vi "Local Error Handler.vi"(6 "Clear? (T)":bool=TRUE, 7 "error in (no error)":errorcluster) -> (9 "error out":errorcluster)   [LabVIEW 2012, in "Win8uiFramework.lvlib"]
uses:
  <vilib>/Utility/error.llb/DialogType.ctl
  Win8uiFramework.lvlib
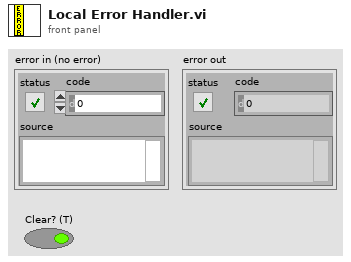
[diagram p1: front panel]
types:
  T1 = typedef "DialogType.ctl" = u16
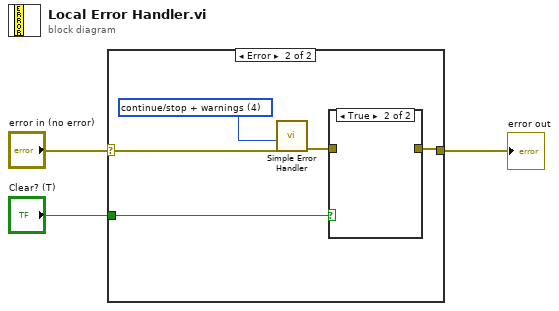
[diagram p0: block diagram]
diagram:
  n1 = case shown="Error" "error in (no error)" {
    selector: "error in (no error)" -> [w4 w9]
    tunnel: [w4 w5] -> w2
    tunnel: "Clear? (T)" -> [_ w6]
    frame No Error {
    }
    frame Error {
      w8 = T1 4 items=["no dialog", "OK message", "continue or stop message", "OK message + warnings", "continue/stop + warnings"] ("type of dialog (OK msg:1)")
      n2 = call <vilib>:"Simple Error Handler.vi"("type of dialog (OK msg:1)"=w8, "error in (no error)"=w9) -> ("error out"=w7:errorcluster)  [unwired: 3 in, 4 out]
      n3 = case shown="True" w6 {
        tunnel: w7 -> [w10 _]
        tunnel: [w10 _] -> w5
        frame False {
        }
        frame True {
        }
      }
    }
  }
  "error out" <- w2
